vi "append1DColumn--timestamp.vi"(6 "Style":refnum<class "Style.lvclass">, 8 "error in (no error)":errorcluster, 10 "Value":timestamp[](array[timestamp]) format="%<%x %.3X>T", 11 "MS-Excel in":refnum<class "MS-Excel.lvclass">) -> (0 "error out":errorcluster, 3 "MS-Excel out":refnum<class "MS-Excel.lvclass">)   [LabVIEW 2017, in "LabVIEW NPOI.lvlib" / "MS-Excel.lvclass"]
uses:
  MS-Excel.lvclass
  Styles/Style/Style.lvclass
  MS-Excel.lvclass/MS-Excel.ctl
  C:/Users/Neo/Desktop/Dev_Tools_BR/LabVIEW_NPOI/lib/NPOI 2.1.1/NPOI.dll
  lib/NPOI 2.1.1/NPOI.dll
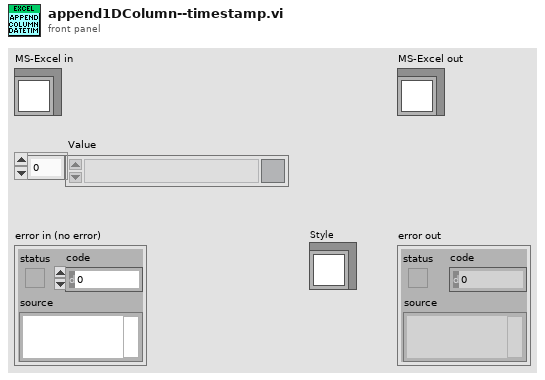
[diagram p1: front panel]
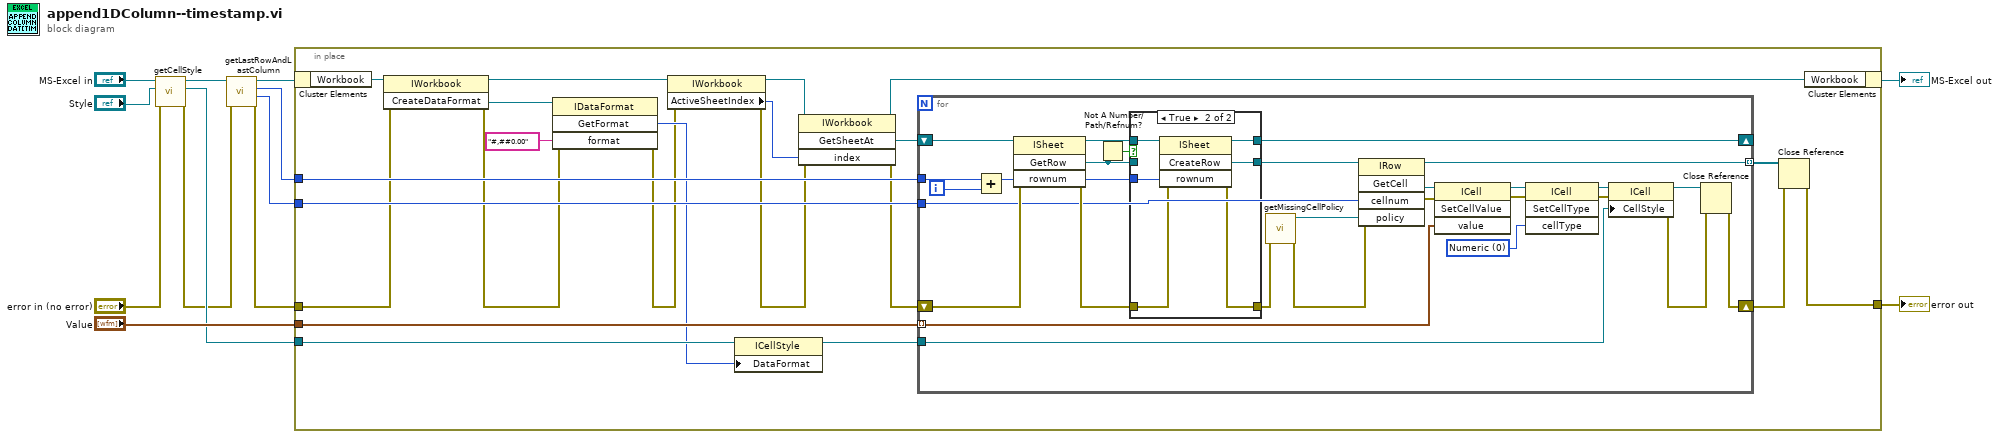
[diagram p0: block diagram]
diagram:
  n1 = call-dynamic "getCellStyle.vi"("error in (no error)"="error in (no error)", "Style"="Style", "MS-Excel in"="MS-Excel in") -> ("error out"=w1:errorcluster, "Cell Style"=w3:refnum<k24>, "MS-Excel out"=w5:refnum<class "MS-Excel.lvclass">)  [unwired: 6 in]
  n2 = call-dynamic "getLastRowAndLastColumn.vi"("error in (no error)"=w1, "MS-Excel in"=w5) -> ("error out"=w8:errorcluster, "Last Column"=w6:i32, "Last Row"=w7:i32, "MS-Excel out"=w9:refnum<class "MS-Excel.lvclass">)  [unwired: 6 in]
  n3 = in-place {
    in-place-border: w8 -> [w15]
    in-place-border: [w30] -> w12
    in-place-border: w7 -> [w35]
    in-place-border: w6 -> [w34]
    in-place-border: "Value" -> [w33]
    in-place-border: w3 -> [w22]
    n4 = in-place-cluster #1(w9) -> ("Workbook"=w23:refnum<k24>)
    n5 = invoke class="IWorkbook" method="CreateDataFormat"(reference=w23, error in=w15) -> (reference out=w21:refnum<k24>, error out=w16:errorcluster, "CreateDataFormat"=w20:refnum<k24>)  [unwired: 1 in]
    n6 = invoke class="IDataFormat" method="GetFormat"(reference=w20, error in=w16, "format"="#,##0.00") -> (error out=w14:errorcluster, "GetFormat"=w17:i16)  [unwired: 1 in, 2 out]
    n7 = property class="IWorkbook"(reference=w21, error in=w14) -> (reference out=w26:refnum<k24>, error out=w24:errorcluster, "ActiveSheetIndex"=w25:i32)
    n8 = property class="ICellStyle"(reference=w22, "DataFormat"=w17) -> (reference out=w18:refnum<k24>)  [unwired: 1 in, 1 out]
    n9 = invoke class="IWorkbook" method="GetSheetAt"(reference=w26, error in=w24, "index"=w25) -> (reference out=w28:refnum<k24>, error out=w27:errorcluster, "GetSheetAt"=w29:refnum<k24>)  [unwired: 1 in, 1 out]
    n10 = for {
      tunnel: w35 -> [w59]
      shift-right: [w58] -> _
      shift-left: w29 -> [w63]
      shift-right: [w50] -> w31
      shift-left: w27 -> [w56]
      tunnel: w34 -> [w36]
      tunnel: w33 -> [w53] mode=indexing
      tunnel: [w49] -> w32 mode=indexing
      tunnel: w18 -> [w44]
      i -> [w48]
      w39 = 0 items=["Numeric"=0, "String"=1, "Formula"=2, "Blank"=3, "Boolean"=4, "Error"=5, "Unknown"=-1] ("cellType")
      n11 = Add(x=w59, y=w48) -> (x+y=w54:i32)
      n12 = invoke class="ISheet" method="GetRow"(reference=w63, error in=w56, "rownum"=w54) -> (reference out=w60:refnum<k24>, error out=w57:errorcluster, "GetRow"=w61:refnum<k24>)  [unwired: 1 in, 1 out]
      n13 = Not A Number/Path/Refnum?(number/path/refnum=w61) -> (NaN/Path/Refnum?=w62:bool)
      n14 = case shown="True" w62 {
        tunnel: w61 -> [w65 _]
        tunnel: w60 -> [w64 w72]
        tunnel: w54 -> [_ w71]
        tunnel: w57 -> [w66 w67]
        tunnel: [w66 w69] -> w46
        tunnel: [w65 w70] -> w55
        tunnel: [w64 w68] -> w58
        frame False {
        }
        frame True {
          n15 = invoke class="ISheet" method="CreateRow"(reference=w72, error in=w67, "rownum"=w71) -> (reference out=w68:refnum<k24>, error out=w69:errorcluster, "CreateRow"=w70:refnum<k24>)  [unwired: 1 in, 1 out]
        }
      }
      n16 = call "getMissingCellPolicy.vi"("error in (no error)"=w46) -> ("error out"=w45:errorcluster, "CREATE_NULL_AS_BLANK"=w47:refnum<k24>)  [unwired: 9 in]
      n17 = invoke class="IRow" method="GetCell"(reference=w55, error in=w45, "cellnum"=w36, "policy"=w47) -> (reference out=w49:refnum<k24>, error out=w42:errorcluster, "GetCell"=w43:refnum<k24>)  [unwired: 1 in, 2 out]
      n18 = invoke class="ICell" method="SetCellValue"(reference=w43, error in=w42, "value"=w53) -> (reference out=w41:refnum<k24>, error out=w40:errorcluster)  [unwired: 1 in, 2 out]
      n19 = invoke class="ICell" method="SetCellType"(reference=w41, error in=w40, "cellType"=w39) -> (reference out=w38:refnum<k24>, error out=w37:errorcluster)  [unwired: 1 in, 2 out]
      n20 = property class="ICell"(reference=w38, error in=w37, "CellStyle"=w44) -> (reference out=w52:refnum<k24>, error out=w51:errorcluster)
      n21 = Close Reference(reference=w52, error in (no error)=w51) -> (error out=w50:errorcluster)
    }
    n22 = Close Reference(reference=w32, error in (no error)=w31) -> (error out=w30:errorcluster)
    n23 = in-place-cluster #1("Workbook"=w28) -> (→"MS-Excel out":refnum<class "MS-Excel.lvclass">)
  }
  "error out" <- w12
